vi "testing_readMeasurements.vi"() -> ()   [LabVIEW 2015, in "Tausand AB1000.lvlib"]
uses:
  <instrlib>/Tausand AB1000/Tausand AB1000.lvlib
  <instrlib>/Tausand AB1000/Public/Controls/deviceTypeRing.ctl
  <vilib>/Analysis/baseanly.llb/Mean (DBL).vi
  <vilib>/Analysis/NI_AALBase.lvlib
panel:
  out "min reading timer (s)":dbl format="%0.4f"
  out "max reading timer (s)":dbl format="%0.4f"
  out "reading timer mean (s)":dbl format="%0.4f"
  out "reading timer histogram":T1(graph)
  in  "stop":bool
  out "last reading timer (s)":dbl format="%0.4f"
  out "error out":errorcluster
  in  "VISA resource name":refnum<visa-resource-name>
  in  "error in (no error)":errorcluster
  out "checksum ok?":bool
  out "read time":timestamp
  out "labels":string[](array[string])
  out "values":u32[](array[numeric])
  in  "read timeout (500 ms)":u32=500
  in  "device type":T2 items=["any"=0, "AB1002"=1002, "AB1004"=1004, "AB1502"=1502, "AB1504"=1504, "AB1902"=1902, "AB1904"=1904, "AB2002"=2002, "AB2004"=2004, "AB2502"=2502, "AB2504"=2504, "AB2902"=2902, "AB2904"=2904]
  # "TEST of: 'Read measurement.vi'"
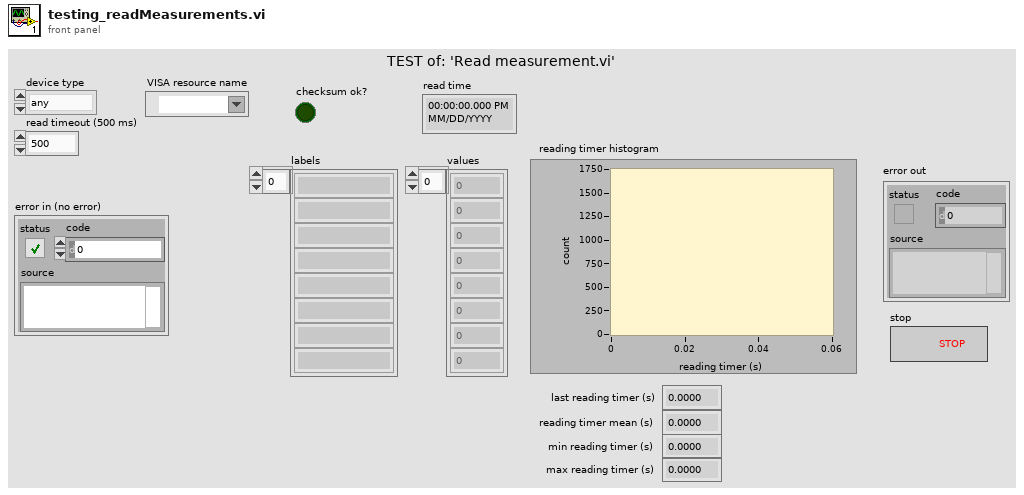
[diagram p1: front panel]
types:
  T1 = cluster{"X Values":dbl[], "Histogram: h(x)":i32[]}
  T2 = typedef "Tausand AB1000.lvlib/deviceTypeRing.ctl" = u16
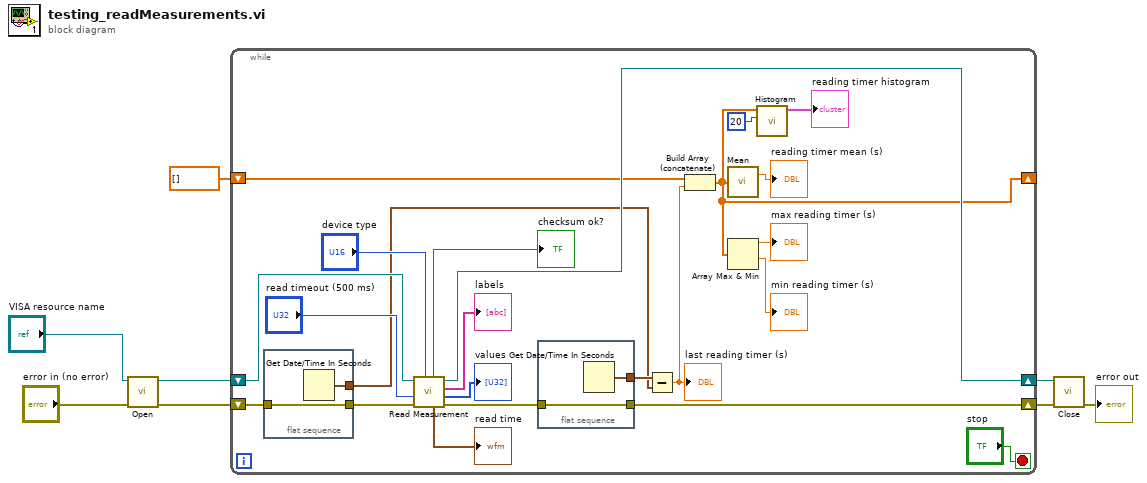
[diagram p0: block diagram]
diagram:
  n1 = call <instrlib>:"Open.vi"("error in (no error)"="error in (no error)", "VISA resource name"="VISA resource name") -> ("error out"=w3:errorcluster, "VISA resource name out"=w8:refnum<visa-resource-name>)  [unwired: 8 in]
  n2 = while {
    shift-right: [w30] -> w7
    shift-left: w8 -> [w31]
    shift-right: [w20] -> w2
    shift-left: w3 -> [w22]
    shift-right: [w11] -> _
    shift-left: dbl[] [] -> [w15]
    stop <- "stop" stop-if-true
    n3 = flat-sequence {
      tunnel: [w35] -> w23
      tunnel: w22 -> [w35]
      tunnel: [w34] -> w18
      frame #0 {
        n4 = Get Date/Time In Seconds() -> (seconds since 1Jan1904=w34:timestamp)
      }
    }
    n5 = call <instrlib>:"Read Measurement.vi"("device type"="device type", "error in (no error)"=w23, "read timeout (500 ms)"="read timeout (500 ms)", "VISA Refnum in"=w31) -> ("error out"=w21:errorcluster, "values"=→"values":u32[], "labels"=→"labels":string[], "VISA Refnum out"=w30:refnum<visa-resource-name>, "read time"=→"read time":timestamp, "checksum ok?"=→"checksum ok?":bool)  [unwired: 2 in]
    n6 = flat-sequence {
      tunnel: [w33] -> w20
      tunnel: w21 -> [w33]
      tunnel: [w32] -> w19
      frame #0 {
        n7 = Get Date/Time In Seconds() -> (seconds since 1Jan1904=w32:timestamp)
      }
    }
    n8 = Subtract(x=w19, y=w18) -> (x-y=w16:dbl)
    "last reading timer (s)" <- w16
    n9 = Build Array (concatenate)(w15, w16) -> (w11:dbl[])
    n10 = call-poly <vilib>:"Mean.vi"("X"=w11) -> ("mean"=→"reading timer mean (s)":dbl)  [unwired: 1 out]
    n11 = Array Max & Min(array=w11) -> (max value=→"max reading timer (s)":dbl, min value=→"min reading timer (s)":dbl)  [unwired: 2 out]
    n12 = call <vilib>:"Histogram.vi"("intervals"=20, "X"=w11) -> ("Histogram Graph"=→"reading timer histogram":T1)  [unwired: 6 in, 3 out]
  }
  n13 = call <instrlib>:"Close.vi"("error in (no error)"=w2, "VISA resource name"=w7) -> ("error out"=→"error out":errorcluster)  [unwired: 9 in]
